vi "Test popup.vi"() -> ()   [LabVIEW 2017]
uses:
  Popup.lvclass
panel:
  in  "Popup":T1 {"Right" items=["High", "Middle", "Low"]}
  in  "多列列表框":i32(listbox)
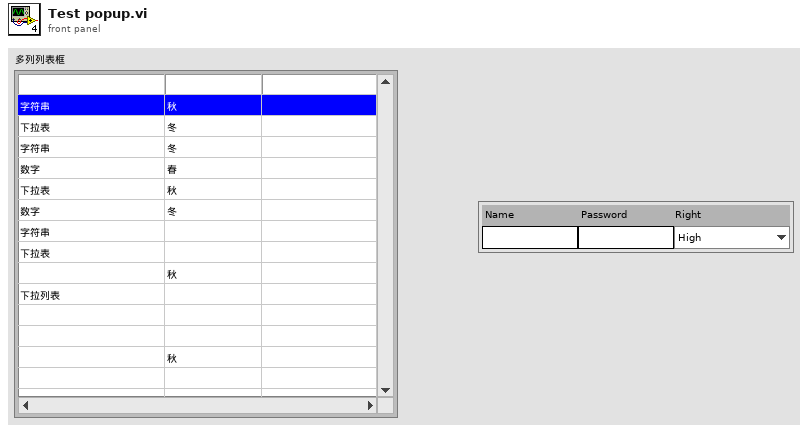
[diagram p1: front panel]
types:
  T1 = cluster{"Name":string, "Password":string, "Right":u16}
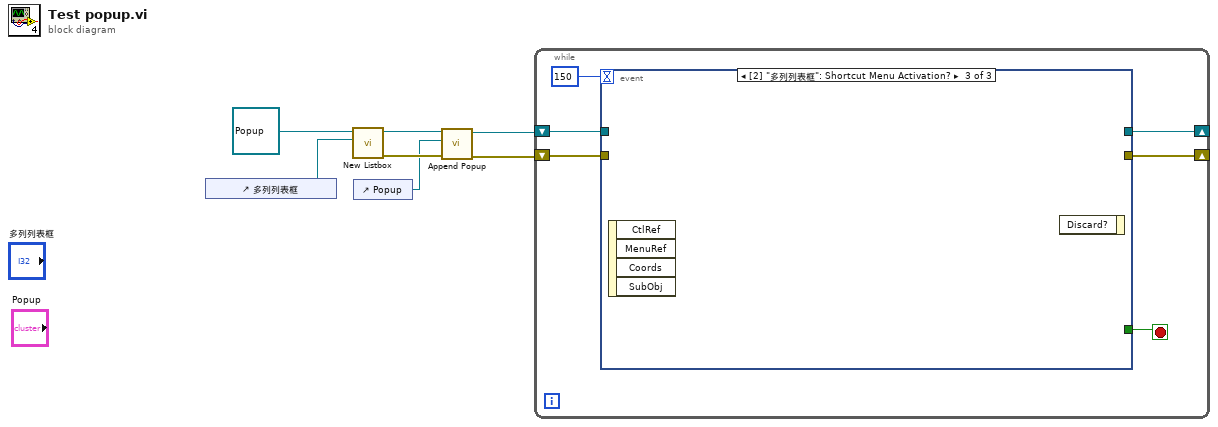
[diagram p0: block diagram]
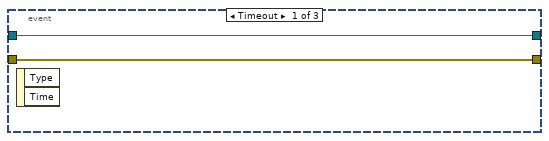
[diagram p2: hidden frame]
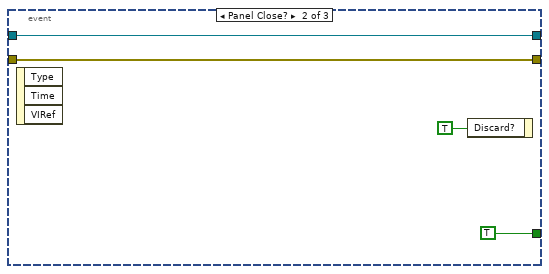
[diagram p3: hidden frame]
diagram:
  n1 = control-ref of="多列列表框"() -> (w6:refnum<vi>)
  n2 = call-dynamic "New Listbox.vi"("ListBox"=w6, "Popup 输入"=refnum<class "Popup.lvclass"> refnum) -> ("error out"=w4:errorcluster, "Popup 输出"=w5:refnum<class "Popup.lvclass">)  [unwired: 8 in]
  n3 = control-ref of="Popup"() -> (w3:refnum<vi>)
  n4 = call-dynamic "Append Popup.vi"("error in (no error)"=w4, "PopupRef"=w3, "Popup 输入"=w5) -> ("error out"=w1:errorcluster, "Popup 输出"=w2:refnum<class "Popup.lvclass">)  [unwired: 7 in]
  n5 = while {
    shift-right: [w11] -> _
    shift-left: w1 -> [w13]
    shift-right: [w10] -> _
    shift-left: w2 -> [w9]
    stop <- w8 stop-if-true
    n6 = event shown="[2] \"多列列表框\": Shortcut Menu Activation?" {
      selector: _ -> [_ _ _]
      dyn-events: _ -> [_ _ _]
      timeout: 150 -> [_ _ _]
      tunnel: w9 -> [w15 w17 _]
      tunnel: w13 -> [w14 w16 _]
      tunnel: [w14 w16 _] -> w11
      tunnel: [w15 w17 _] -> w10
      tunnel: [_ TRUE _] -> w8
      event Timeout {
        n7 = event-data() -> ()  [unwired: 1 in, 2 out]
      }
      event Panel Close? {
        n8 = event-data() -> ()  [unwired: 1 in, 3 out]
        n9 = event-data("Discard?"=TRUE) -> ()  [unwired: 1 in, 1 out]
      }
      event "多列列表框": Shortcut Menu Activation? {
        n10 = event-data() -> ()  [unwired: 1 in, 4 out]
        n11 = event-data() -> ()  [unwired: 2 in, 1 out]
      }
    }
  }
